vi "trace_property_stringSet_sub.vi"(0 "char nr max":i32[](array[numeric]), 5 "trace idx global":u32, 7 "parameter_name":string[](array[string]), 9 "parameter_value":string, 11 "error in (no error)":errorcluster) -> (15 "error out":errorcluster)   [LabVIEW 2010, in "OSA.lvclass"]
uses:
  OSA.lvclass
  FTSLib.dll
  OSA20X_misc.lvlib
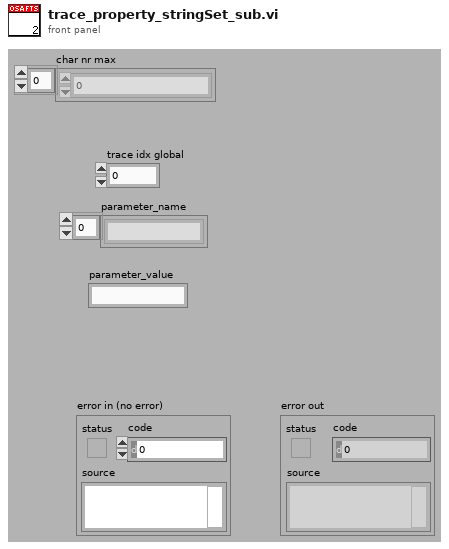
[diagram p1: front panel]
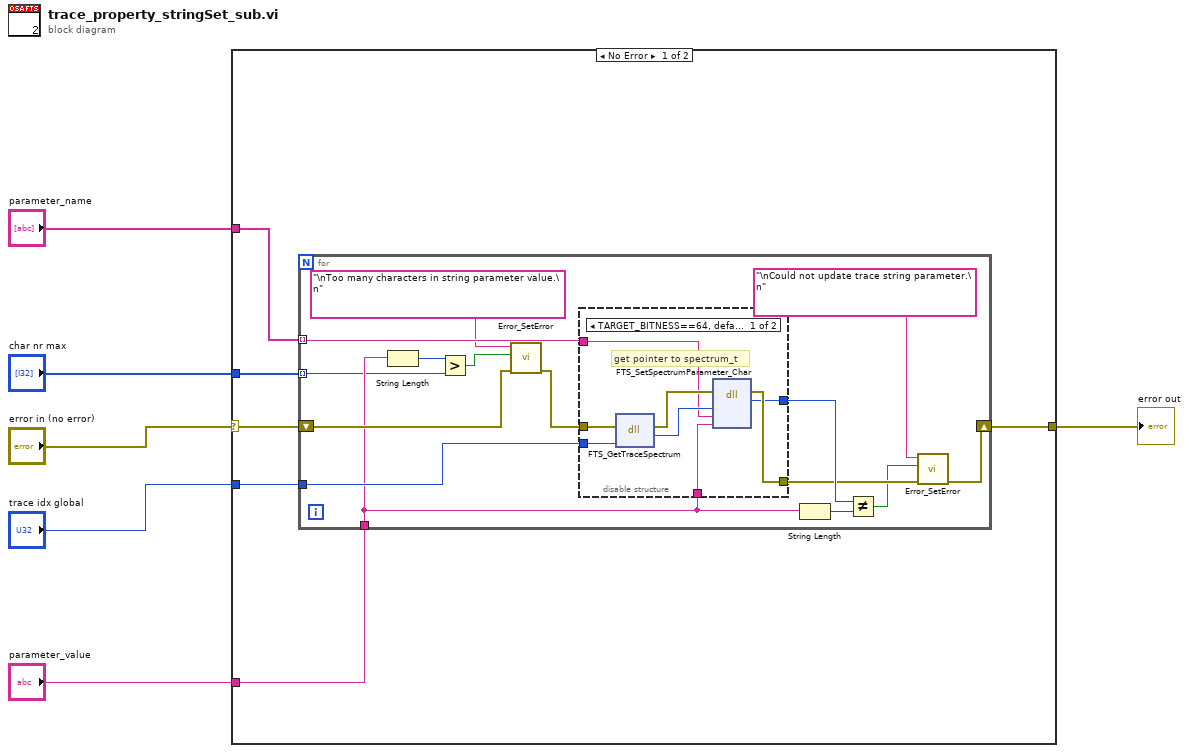
[diagram p0: block diagram]
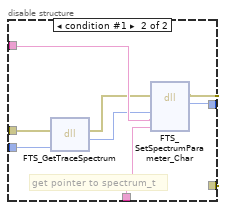
[diagram p2: hidden frame]
diagram:
  n1 = case shown="No Error" "error in (no error)" {
    selector: "error in (no error)" -> [w7 w44]
    tunnel: "parameter_name" -> [w12 _]
    tunnel: "trace idx global" -> [w10 _]
    tunnel: [w11 w44] -> w4
    tunnel: "parameter_value" -> [w9 _]
    tunnel: "char nr max" -> [w8 _]
    frame No Error {
      n2 = for {
        tunnel: w10 -> [w20]
        shift-right: [w22] -> w11
        shift-left: w7 -> [w16]
        tunnel: w12 -> [w27] mode=indexing
        tunnel: w9 -> [w14]
        tunnel: w8 -> [w13] mode=indexing
        n3 = String Length(string=w14) -> (length=w17:i32)
        n4 = Greater?(x=w17, y=w13) -> (0:w18:bool)
        n5 = call "Error_SetError.vi"("error in"=w16, "status (true)"=w18, "source(\"\")"="\nToo many characters in string parameter value.\n" ("source(\"\")")) -> ("error out"=w15:errorcluster)  [unwired: 4 in]
        n6 = disable-structure shown="TARGET_BITNESS==64, default" {
          disable-tunnel: w20 -> [w35 w42]
          disable-tunnel: w15 -> [w32 w43]
          disable-tunnel: [w31 w39] -> w24
          disable-tunnel: w27 -> [w29 w41]
          disable-tunnel: [w30 w37] -> w25
          disable-tunnel: w14 -> [w28 w36]
          frame condition #0 (active) {
            # "get pointer to spectrum_t"
            n7 = dll-call lib="FTSLib.dll" fn="FTS_GetTraceSpectrum"(error in=w32, "traceIdx"=w35) -> (error out=w33:errorcluster, "spectrum_t_pointer"=w34:u64)  [unwired: 3 in, 1 out]
            n8 = dll-call lib="FTSLib.dll" fn="FTS_SetSpectrumParameter_Char"(error in=w33, "spectrum_t_pointer"=w34, "parameter_name"=w29, "parameter_value"=w28) -> (error out=w31:errorcluster, "return"=w30:i32)  [unwired: 5 in, 1 out]
          }
          frame condition #1 {
            # "get pointer to spectrum_t"
            n9 = dll-call lib="FTSLib.dll" fn="FTS_GetTraceSpectrum"(error in=w43, "traceIdx"=w42) -> (error out=w40:errorcluster, "spectrum_t_pointer"=w38:u32)  [unwired: 3 in, 1 out]
            n10 = dll-call lib="FTSLib.dll" fn="FTS_SetSpectrumParameter_Char"(error in=w40, "spectrum_t_pointer"=w38, "parameter_name"=w41, "parameter_value"=w36) -> (error out=w39:errorcluster, "return"=w37:i32)  [unwired: 5 in, 1 out]
          }
        }
        n11 = String Length(string=w14) -> (length=w26:i32)
        n12 = Not Equal?(x=w25, y=w26) -> (x != y?=w23:bool)
        n13 = call "Error_SetError.vi"("error in"=w24, "status (true)"=w23, "source(\"\")"="\nCould not update trace string parameter.\n" ("source(\"\")")) -> ("error out"=w22:errorcluster)  [unwired: 4 in]
      }
    }
    frame Error {
    }
  }
  "error out" <- w4
